vi "Write Array of Observers.vi"(8 "error in (no error)":errorcluster, 10 "Array of Observers":refnum<class "Send.lvclass">[](array[class]), 11 "ObserverSet.lvclass in":refnum<class "ObserverSet.lvclass">) -> (0 "error out":errorcluster, 3 "ObserverSet.lvclass out":refnum<class "ObserverSet.lvclass">)   [LabVIEW 2011, in "Messenging.lvlib" / "ObserverSet.lvclass"]
uses:
  ObserverSet.lvclass
  Send/Send.lvclass
  ObserverSet.lvclass/ObserverSet.ctl
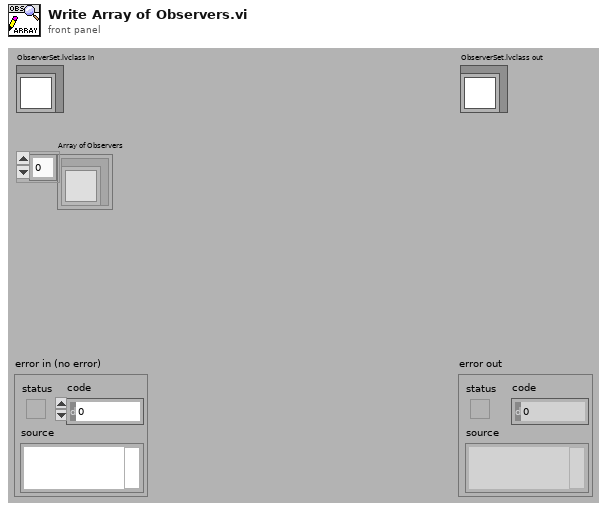
[diagram p1: front panel]
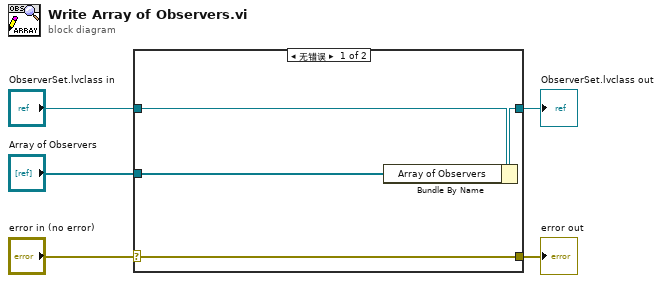
[diagram p0: block diagram]
diagram:
  n1 = case shown="无错误" "error in (no error)" {
    selector: "error in (no error)" -> [w9 w10]
    tunnel: [w9 w10] -> w4
    tunnel: [w7 w11] -> w2
    tunnel: "ObserverSet.lvclass in" -> [w8 w11]
    tunnel: "Array of Observers" -> [w6 _]
    frame No Error {
      n2 = Bundle By Name(cluster=w8, "Array of Observers"=w6) -> (w7:refnum<class "ObserverSet.lvclass">)
    }
    frame Error {
    }
  }
  "error out" <- w4
  "ObserverSet.lvclass out" <- w2
